vi "test harness_FXP_L_ye_Bend_u_singleAxis_REAL_DATA.vi"(8 "error in (no error)":errorcluster, 11 "TestCase in":refnum<class "FXP_observer_TestCase.lvclass">) -> (0 "error out":errorcluster, 3 "TestCase out":refnum<class "FXP_observer_TestCase.lvclass">)   [LabVIEW 2019, in "FXP_observer_TestCase.lvclass"]
uses:
  FXP_observer_TestCase.lvclass
  <vilib>/rvi/DesktopExecutionNode/Execution/niFpgaDEN_Execute.vi
  <vilib>/rvi/DesktopExecutionNode/DesktopExecutionNode.xnode
  <vilib>/addons/_JKI Toolkits/VI Tester/TestCase.llb/TestCase.lvclass
  C:/Program Files (x86)/National Instruments/LabVIEW 2019/vi.lib/addons/_JKI Toolkits/VI Tester/TestCase.llb/TestCase.lvclass
panel:
  out "x+y":fxp<+/-,51,11>[](array[numeric])
  out "xk_1_1":fxp<+/-,32,5>[](array[numeric])
  out "error (x_1_1)":errorcluster
  out "error (xu)":errorcluster
  out "error (yd)":errorcluster
  in  "U(k): ux":fxp<+/-,18,5>=0.14501953125
  in  "y(k)":fxp<+/-,18,5>=0.123046875
  # "Remember that Ldist and Bz only have\ntwo integer bits!"
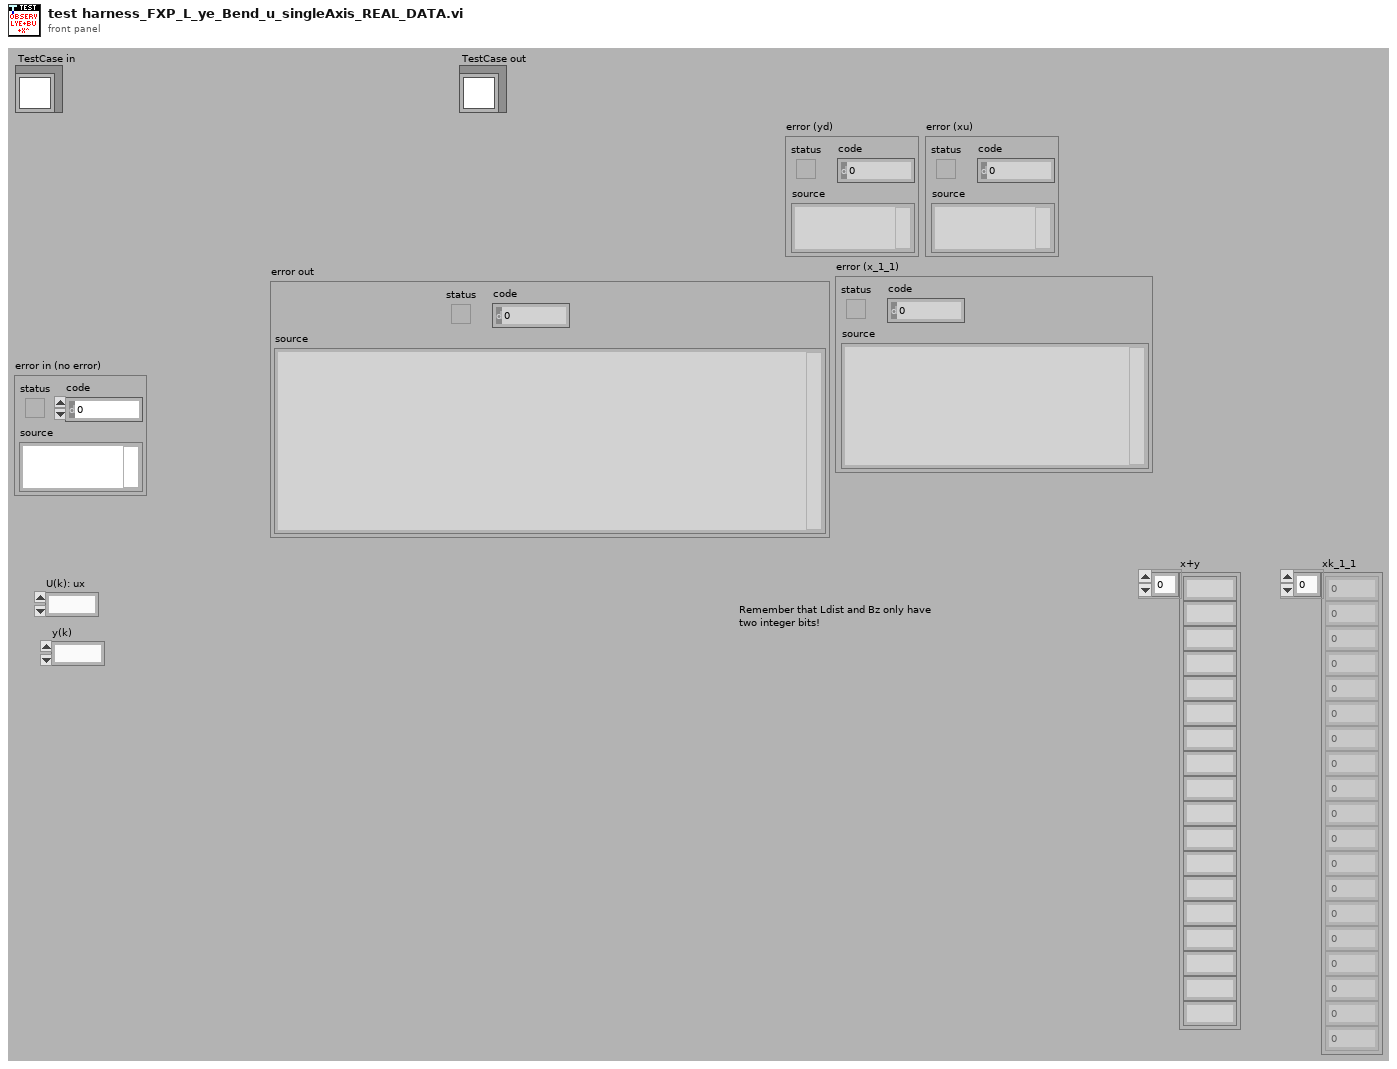
[diagram p1: front panel]
types:
  T1 = typedef "UT_matrix_data.ctl" = cluster{"Bz":T2[], "Ldist":T3[], "Kz":T4[], "Nx":T5[], "Ax_col":T6[], "X_vec":T7[], "Cz":T8[]}
  T2 = typedef "Bz_vec_scalar.ctl" = fxp<+/-,32,3>
  T3 = typedef "Lz_vec_scalar.ctl" = fxp<+/-,32,3>
  T4 = typedef "Kz_vec_scalar.ctl" = fxp<+/-,32,10>
  T5 = typedef "Nx_vec_scalar.ctl" = fxp<+/-,32,2>
  T6 = typedef "Az_vec_scalar.ctl" = fxp<+/-,32,7>
  T7 = typedef "x_vec_scalar.ctl" = fxp<+/-,32,6>
  T8 = typedef "Cz_vec_scalar.ctl" = fxp<+/-,32,4>
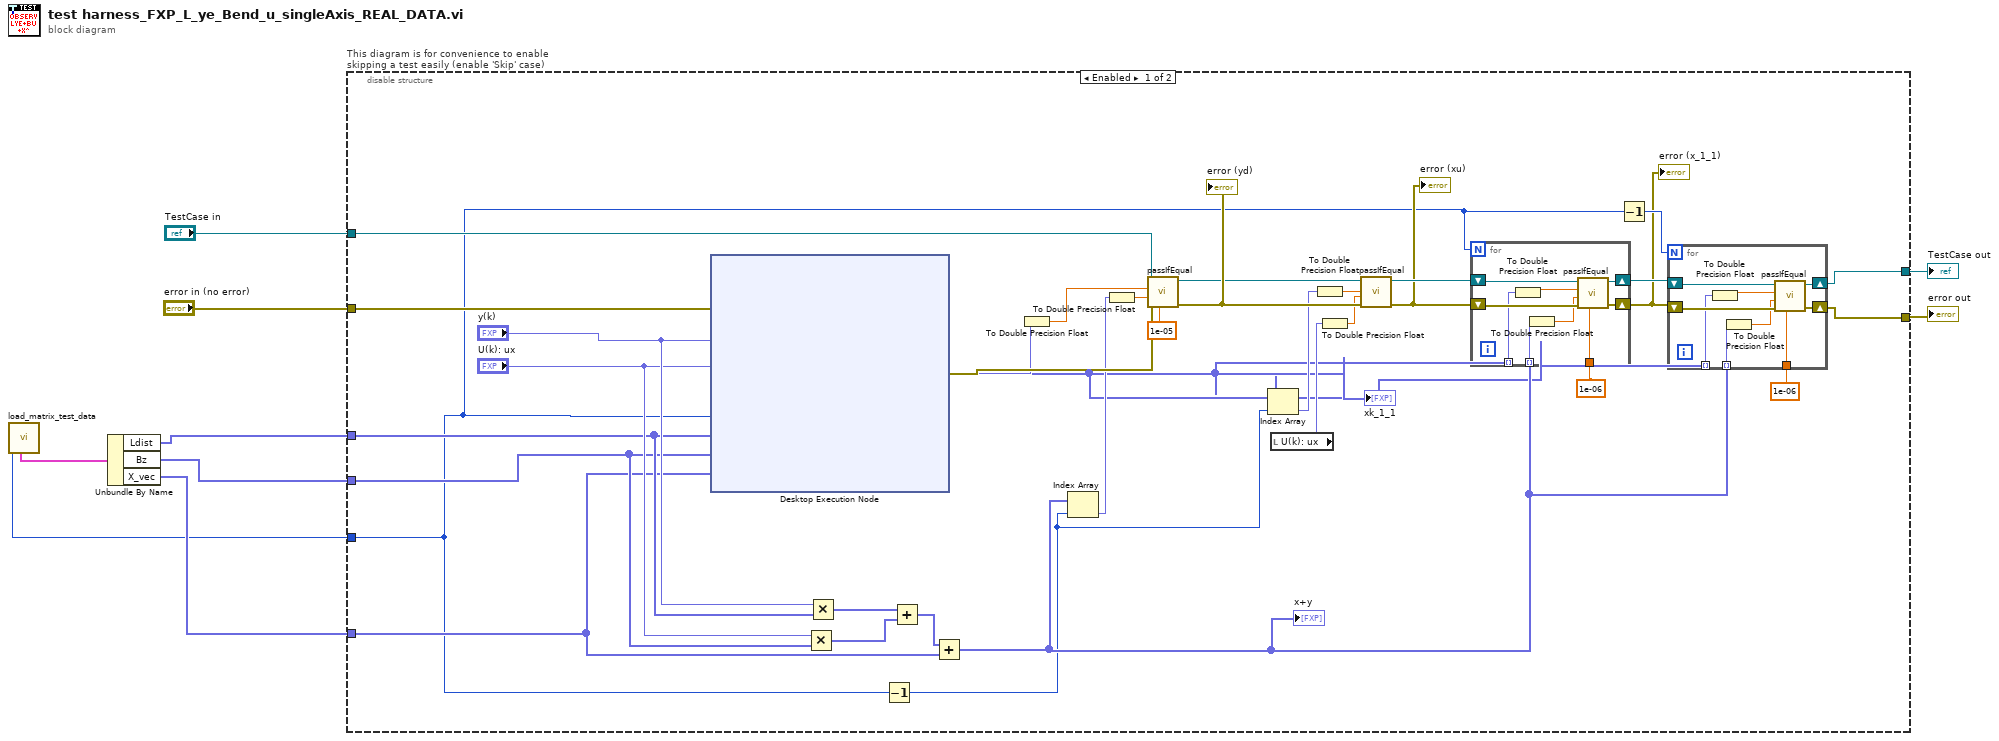
[diagram p0: block diagram]
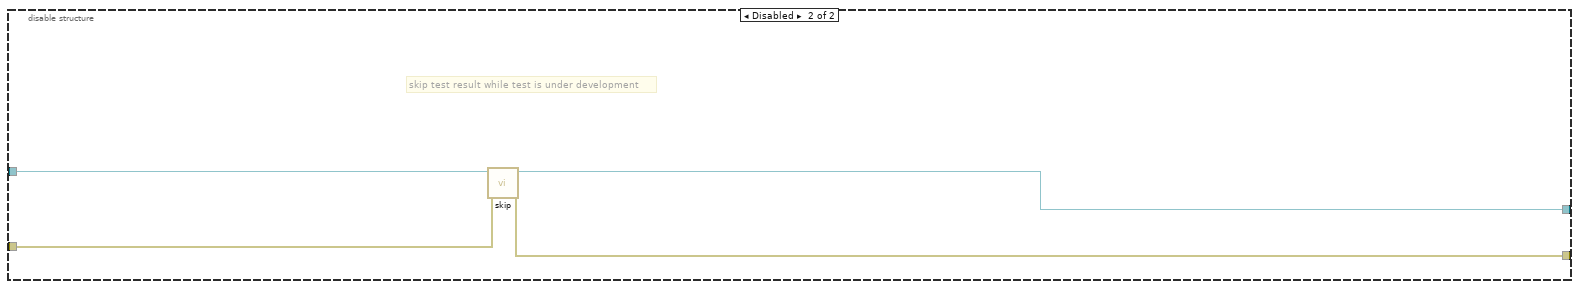
[diagram p2: hidden frame]
diagram:
  n1 = call "load_matrix_test_data.vi"() -> ("output cluster"=w5:T1, "Ns"=w1:i32)  [unwired: 4 in, 6 out]
  n2 = Unbundle By Name(w5) -> ("Ldist"=w4:T3[], "Bz"=w3:T2[], "X_vec"=w2:T7[])
  n3 = disable-structure "This diagram is for convenience to enable skipping a test easily (enable 'Skip' case)" shown="Enabled" {
    disable-tunnel: "TestCase in" -> [w45 w67]
    disable-tunnel: [w22 w65] -> w6
    disable-tunnel: [w21 w66] -> w8
    disable-tunnel: "error in (no error)" -> [w41 w64]
    disable-tunnel: w4 -> [w14 _]
    disable-tunnel: w3 -> [w13 _]
    disable-tunnel: w2 -> [w12 _]
    disable-tunnel: w1 -> [w10 _]
    frame Enabled {
      n4 = xnode "Desktop Execution Node"("Error In"=w41, "y(k)"="y(k)", "U(k): ux"="U(k): ux", "NS"=w10, "Ldist"=w14, "Bz"=w13, "x"=w12) -> ("Error Out"=w42:errorcluster, "yd_est"=w35:fxp<+/-,32,5>, "xk_1_1"=w25:fxp<+/-,32,5>[], "xk_1_2"=w17:fxp<+/-,32,5>[])
      "xk_1_1" <- w25
      n5 = Multiply(x="U(k): ux", y=w13) -> (x*y=w37:fxp<+/-,50,8>[])
      n6 = Multiply(x="y(k)", y=w14) -> (x*y=w38:fxp<+/-,50,8>[])
      n7 = Decrement(x=w10) -> (x-1=w11:i32)
      n8 = Add(x=w38, y=w37) -> (x+y=w36:fxp<+/-,51,9>[])
      n9 = Add(x=w36, y=w12) -> (x+y=w18:fxp<+/-,51,9>[])
      "x+y" <- w18
      n10 = To Double Precision Float(number=w35) -> (double precision float=w43:dbl)
      n11 = Index Array(array=w18, index=w11) -> (element=w33:fxp<+/-,51,9>)
      n12 = To Double Precision Float(number=w33) -> (double precision float=w34:dbl)
      n13 = call-dynamic "passIfEqual.vi"("delta (optional)"=1e-05 ("del u_x"), "error in (no error)"=w42, "y"=w34, "x"=w43, "TestCase in"=w45) -> ("error out"=w32:errorcluster, "TestCase out"=w31:refnum<class "FXP_observer_TestCase.lvclass">)  [unwired: 5 in]
      "error (yd)" <- w32
      n14 = Index Array(array=w17, index=w11) -> (element=w29:fxp<+/-,32,5>)
      n15 = local read "U(k): ux"() -> (w27:fxp<+/-,18,5>)
      n16 = To Double Precision Float(number=w29) -> (double precision float=w30:dbl)
      n17 = To Double Precision Float(number=w27) -> (double precision float=w28:dbl)
      n18 = call-dynamic "passIfEqual.vi"("error in (no error)"=w32, "y"=w28, "x"=w30, "TestCase in"=w31) -> ("error out"=w16:errorcluster, "TestCase out"=w26:refnum<class "FXP_observer_TestCase.lvclass">)  [unwired: 6 in]
      "error (xu)" <- w16
      n19 = for {
        N: w10 -> [_]
        shift-right: [w63] -> w23
        shift-left: w26 -> [w60]
        shift-right: [w62] -> w15
        shift-left: w16 -> [w61]
        tunnel: w18 -> [w59] mode=indexing
        tunnel: w25 -> [w56] mode=indexing
        tunnel: 1e-06 ("del u_x") -> [w55]
        n20 = To Double Precision Float(number=w56) -> (double precision float=w57:dbl)
        n21 = To Double Precision Float(number=w59) -> (double precision float=w58:dbl)
        n22 = call-dynamic "passIfEqual.vi"("delta (optional)"=w55, "error in (no error)"=w61, "y"=w58, "x"=w57, "TestCase in"=w60) -> ("error out"=w62:errorcluster, "TestCase out"=w63:refnum<class "FXP_observer_TestCase.lvclass">)  [unwired: 5 in]
      }
      "error (x_1_1)" <- w15
      n23 = Decrement(x=w10) -> (x-1=w19:i32)
      n24 = for {
        N: w19 -> [_]
        shift-right: [w54] -> w22
        shift-left: w23 -> [w51]
        shift-right: [w53] -> w21
        shift-left: w15 -> [w52]
        tunnel: w18 -> [w50] mode=indexing
        tunnel: w17 -> [w47] mode=indexing
        tunnel: 1e-06 ("del u_x") -> [w46]
        n25 = To Double Precision Float(number=w47) -> (double precision float=w48:dbl)
        n26 = To Double Precision Float(number=w50) -> (double precision float=w49:dbl)
        n27 = call-dynamic "passIfEqual.vi"("delta (optional)"=w46, "error in (no error)"=w52, "y"=w49, "x"=w48, "TestCase in"=w51) -> ("error out"=w53:errorcluster, "TestCase out"=w54:refnum<class "FXP_observer_TestCase.lvclass">)  [unwired: 5 in]
      }
    }
    frame Disabled {
      # "skip test result while test is under development"
      n28 = call <vilib>:"skip.vi"("error in (no error)"=w64, "TestCase in"=w67) -> ("error out"=w66:errorcluster, "TestCase out"=w65:refnum<class "FXP_observer_TestCase.lvclass">)  [unwired: 8 in]
    }
  }
  "error out" <- w8
  "TestCase out" <- w6
